vi "H3C psw cable 10G SFP+读写操作.vi"(6 "input_psw":u8[](array[numeric]) format="%.0x", 7 "input_psw 2":u8[](array[numeric]) format="%.0x", 8 "input_data":u8[](array[numeric]) format="%.0x", 9 "input_mode":string(combo), 10 "Channel":u8 max=5 step=1, 11 "VISA":refnum<visa-resource-name>="COM6") -> (0 "A2Hequal00?":bool, 1 "result":bool, 2 "message":string, 3 "data read":u8[](array[numeric]) format="%.0x")   [LabVIEW 2011]
panel:
  out "A2h后128个字节":u8[](array[numeric]) format="%.0x"
  out "A2h前128个字节":u8[](array[numeric]) format="%.0x"
  in  "address":u8
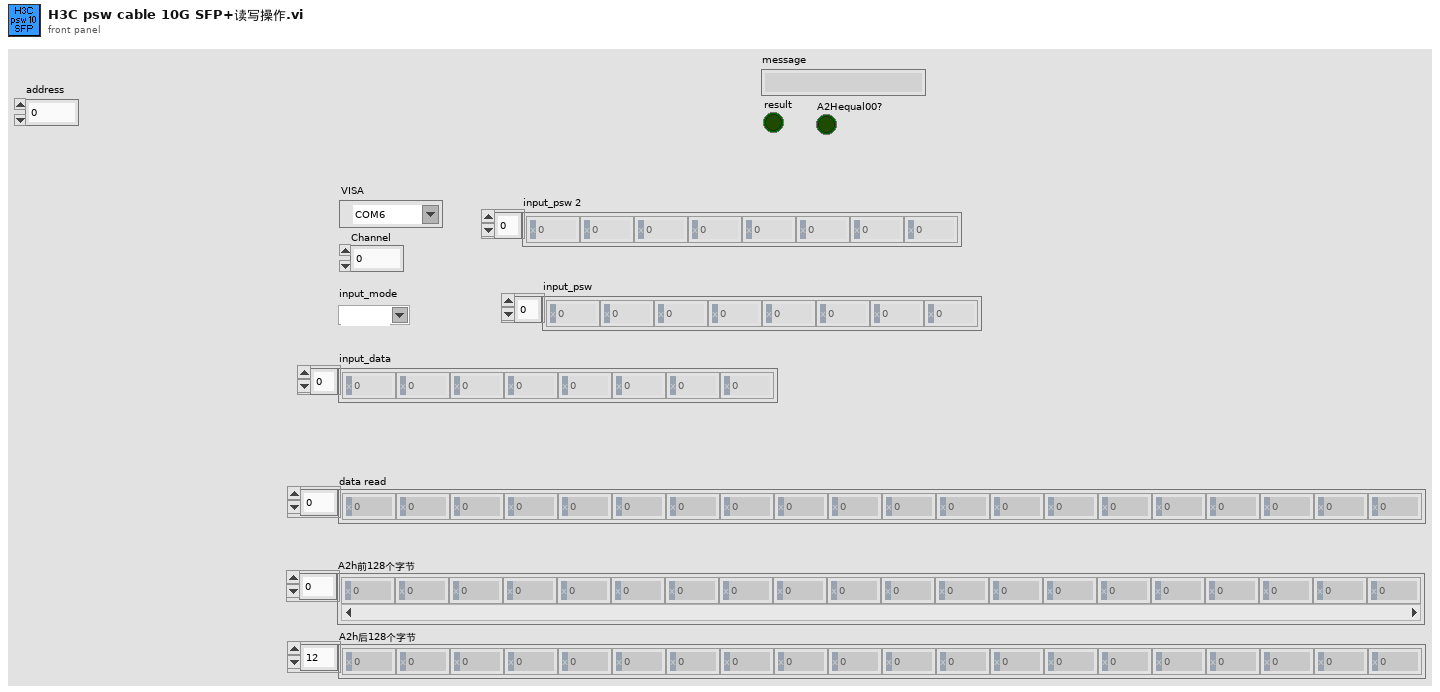
[diagram p1: front panel]
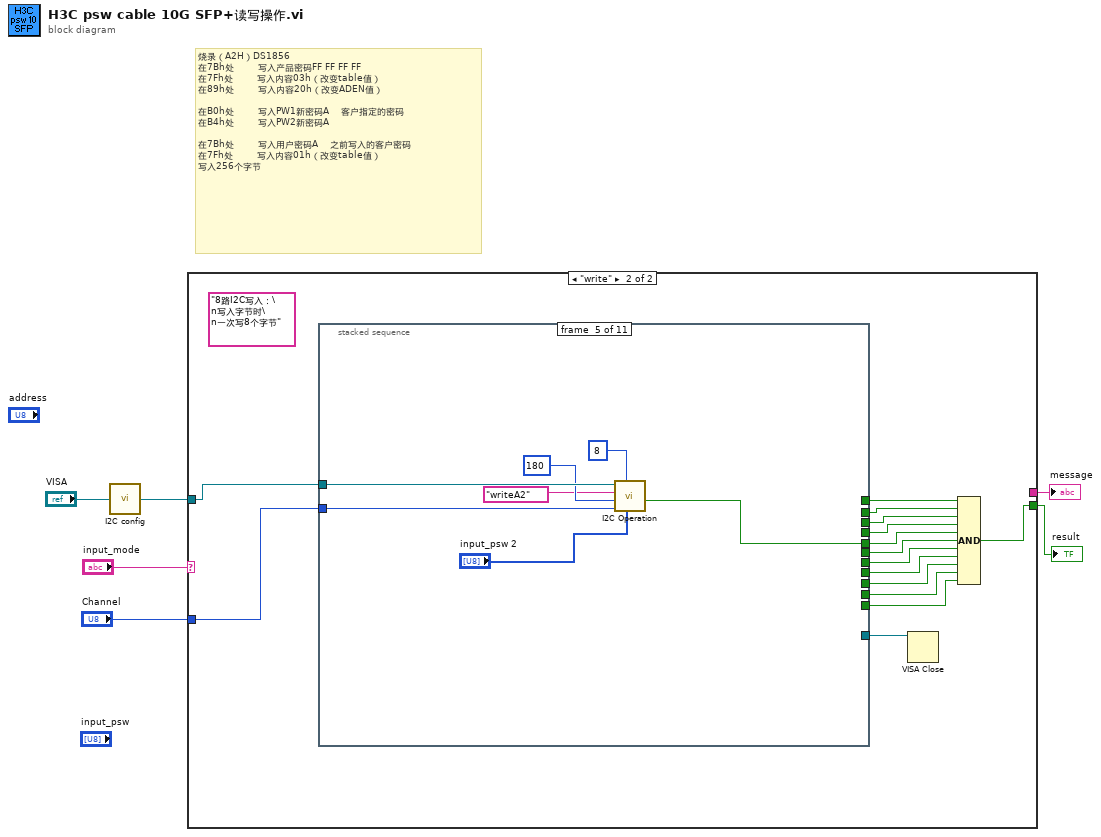
[diagram p0: block diagram]
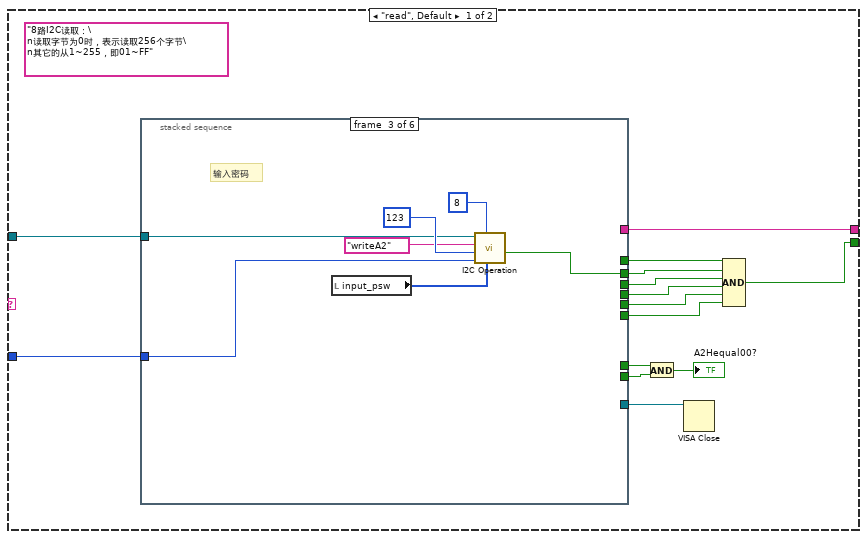
[diagram p2: hidden frame]
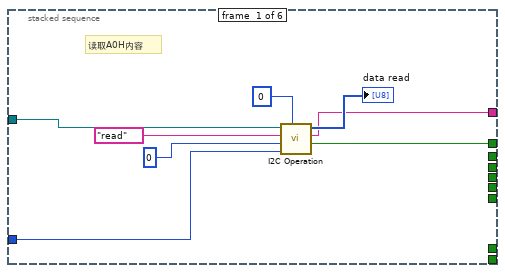
[diagram p3: hidden frame]
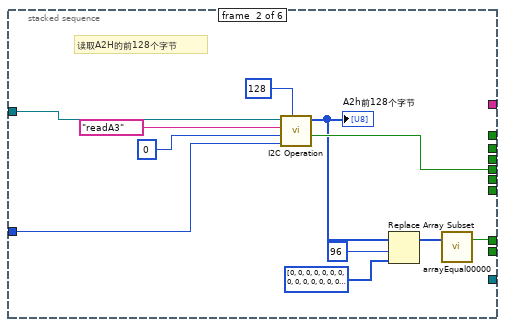
[diagram p4: hidden frame]
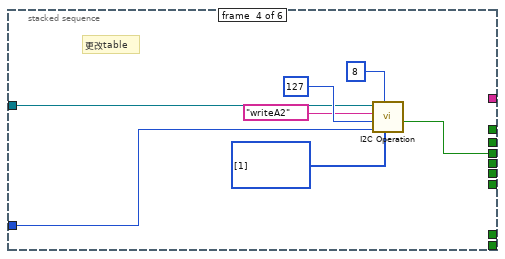
[diagram p5: hidden frame]
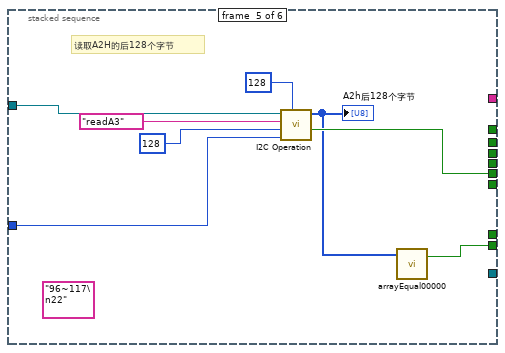
[diagram p6: hidden frame]
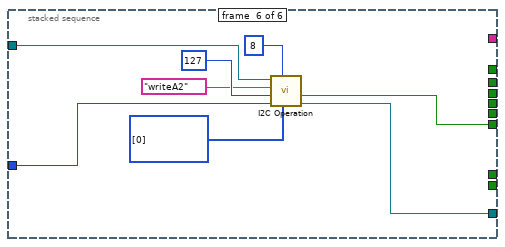
[diagram p7: hidden frame]
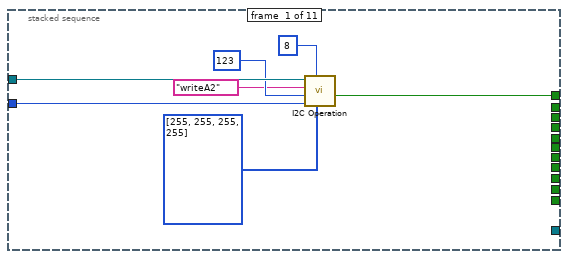
[diagram p8: hidden frame]
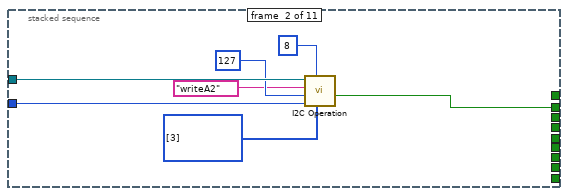
[diagram p9: hidden frame]
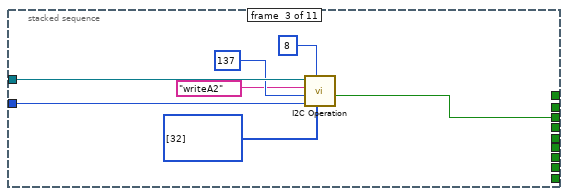
[diagram p10: hidden frame]
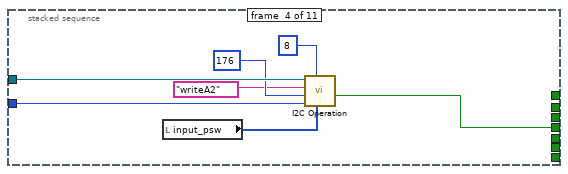
[diagram p11: hidden frame]
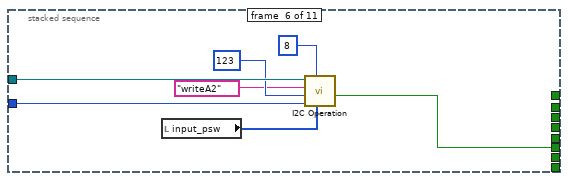
[diagram p12: hidden frame]
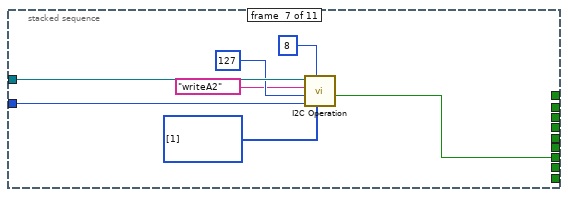
[diagram p13: hidden frame]
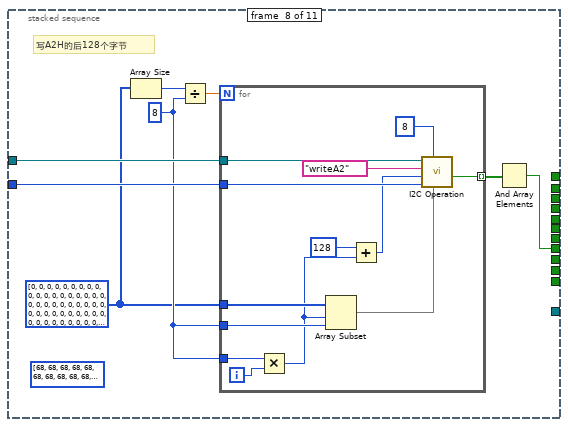
[diagram p14: hidden frame]
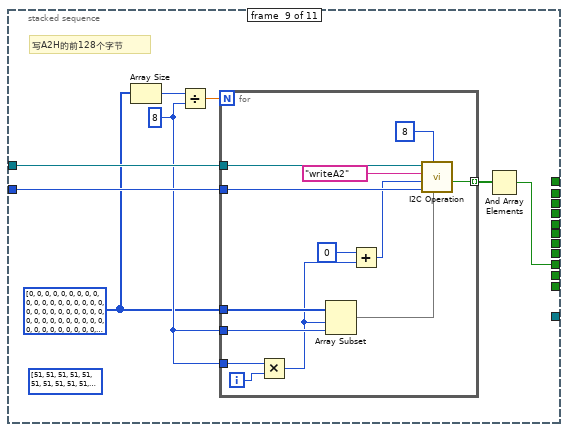
[diagram p15: hidden frame]
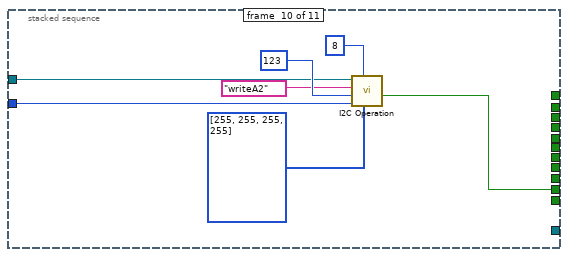
[diagram p16: hidden frame]
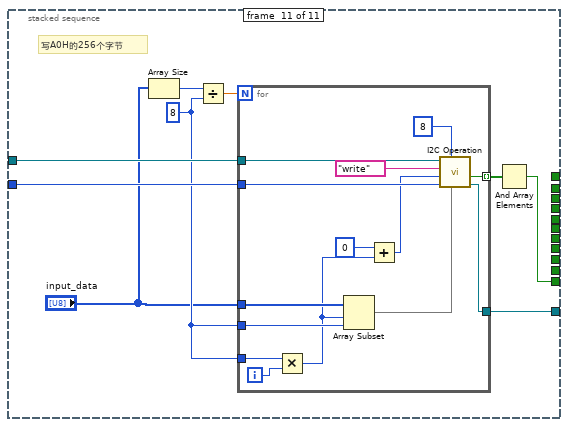
[diagram p17: hidden frame]
diagram:
  # "烧录（A2H）DS1856\n在7Bh处        写入产品密码FF FF FF FF\n在7Fh处        写入内容03h（改变table值）\n在89h处        写入内容20h（改变ADEN值）\n\n在B0h处        写入PW1新密码A    客户指定的密码\n在B4h处        写入PW2新密码A\n\n在7Bh处        写入用户密码A    之前写入的客户密码\n在7Fh处        写入内容01h（改变table值）\n写入256个字节"
  n1 = call "I2C config.vi"("VISA"="VISA") -> ("VISA资源名称输出"=w1:refnum<visa-resource-name>)
  n2 = case shown="\"write\"" "input_mode" {
    tunnel: w1 -> [w20 w84]
    tunnel: "Channel" -> [w19 w83]
    tunnel: [w18 _] -> w4
    tunnel: [w12 w71] -> w3
    frame "read", Default {
      (unwired) "8路I2C读取：\n读取字节为0时，表示读取256个字节\n其它的从1~255，即01~FF"
      n3 = stacked-sequence {
        tunnel: w20 -> [w28 w39 w42 w49 w61 w65]
        tunnel: w19 -> [w25 w36 w41 w48 w58 w64]
        tunnel: [w23 _ _ _ _ _] -> w18
        tunnel: [w22 _ _ _ _ _] -> w17
        tunnel: [_ _ w40 _ _ _] -> w16
        tunnel: [_ _ _ w47 _ _] -> w15
        tunnel: [_ w34 _ _ _ _] -> w14
        tunnel: [_ w33 _ _ _ _] -> w11
        tunnel: [_ _ _ _ w56 _] -> w13
        tunnel: [_ _ _ _ w55 _] -> w10
        tunnel: [_ _ _ _ _ w63] -> w8
        tunnel: [_ _ _ _ _ w62] -> w7
        frame #0 {
          # "读取A0H内容"
          n4 = call "I2C Operation.vi"("size"=0, "Channel"=w25, "address"=u8 0, "mode"="read", "VISA"=w28) -> ("result"=w22:bool, "message"=w23:string, "Data Out"=→"data read":u8[])  [unwired: 3 in, 1 out]
        }
        frame #1 {
          # "读取A2H的前128个字节"
          n5 = call "I2C Operation.vi"("size"=128, "Channel"=w36, "address"=u8 0, "mode"="readA3", "VISA"=w39) -> ("result"=w34:bool, "Data Out"=w29:u8[])  [unwired: 3 in, 2 out]
          "A2h前128个字节" <- w29
          n6 = Replace Array Subset(array=w29, new element=u8[] [0, 0, 0, 0, 0, 0, 0, 0, 0, 0, 0, 0, 0, 0, 0, 0, 0, 0, 0, 0, 0, 0], index=96 ("索引")) -> (w30:u8[])
          n7 = call "arrayEqual00000.vi"("input_array"=w30) -> ("show_bool_result"=w33:bool)  [unwired: 2 in]
        }
        frame #2 {
          # "输入密码"
          n8 = local read "input_psw"() -> (w44:u8[])
          n9 = call "I2C Operation.vi"("input_data"=w44, "size"=8, "Channel"=w41, "address"=u8 123, "mode"="writeA2", "VISA"=w42) -> ("result"=w40:bool)  [unwired: 2 in, 3 out]
        }
        frame #3 {
          # "更改table"
          n10 = call "I2C Operation.vi"("input_data"=u8[] [1], "size"=8, "Channel"=w48, "address"=u8 127, "mode"="writeA2", "VISA"=w49) -> ("result"=w47:bool)  [unwired: 2 in, 3 out]
        }
        frame #4 {
          (unwired) "96~117\n22"
          # "读取A2H的后128个字节"
          n11 = call "I2C Operation.vi"("size"=128, "Channel"=w58, "address"=u8 128, "mode"="readA3", "VISA"=w61) -> ("result"=w56:bool, "Data Out"=w54:u8[])  [unwired: 3 in, 2 out]
          "A2h后128个字节" <- w54
          n12 = call "arrayEqual00000.vi"("input_array"=w54) -> ("show_bool_result"=w55:bool)  [unwired: 2 in]
        }
        frame #5 {
          n13 = call "I2C Operation.vi"("input_data"=u8[] [0], "size"=8, "Channel"=w64, "address"=u8 127, "mode"="writeA2", "VISA"=w65) -> ("VISA  2"=w62:refnum<visa-resource-name>, "result"=w63:bool)  [unwired: 2 in, 2 out]
        }
      }
      n14 = And(x=w11, y=w10) -> (x .and. y?=→"A2Hequal00?":bool)
      n15 = VISA Close(VISA resource name=w7) -> ()  [unwired: 1 in, 1 out]
      n16 = Compound Arithmetic op=AND(w17, w16, w15, w14, w13, w8) -> (w12:bool)
    }
    frame "write" {
      (unwired) "8路I2C写入：\n写入字节时\n一次写8个字节"
      n17 = stacked-sequence {
        tunnel: w84 -> [w91 w98 w105 w112 w119 w126 w133 w141 w162 w179 w191]
        tunnel: w83 -> [w89 w96 w103 w110 w117 w124 w131 w140 w161 w178 w190]
        tunnel: [w85 _ _ _ _ _ _ _ _ _ _] -> w82
        tunnel: [_ w92 _ _ _ _ _ _ _ _ _] -> w81
        tunnel: [_ _ w99 _ _ _ _ _ _ _ _] -> w80
        tunnel: [_ _ _ w106 _ _ _ _ _ _ _] -> w79
        tunnel: [_ _ _ _ w114 _ _ _ _ _ _] -> w78
        tunnel: [_ _ _ _ _ w120 _ _ _ _ _] -> w77
        tunnel: [_ _ _ _ _ _ w127 _ _ _ _] -> w76
        tunnel: [_ _ _ _ _ _ _ w135 _ _ _] -> w75
        tunnel: [_ _ _ _ _ _ _ _ w156 _ _] -> w74
        tunnel: [_ _ _ _ _ _ _ _ _ w176 _] -> w73
        tunnel: [_ _ _ _ _ _ _ _ _ _ w185] -> w72
        tunnel: [_ _ _ _ _ _ _ _ _ _ w183] -> w70
        frame #0 {
          n18 = call "I2C Operation.vi"("input_data"=u8[] [255, 255, 255, 255], "size"=8, "Channel"=w89, "address"=u8 123, "mode"="writeA2", "VISA"=w91) -> ("result"=w85:bool)  [unwired: 2 in, 3 out]
        }
        frame #1 {
          n19 = call "I2C Operation.vi"("input_data"=u8[] [3], "size"=8, "Channel"=w96, "address"=u8 127, "mode"="writeA2", "VISA"=w98) -> ("result"=w92:bool)  [unwired: 2 in, 3 out]
        }
        frame #2 {
          n20 = call "I2C Operation.vi"("input_data"=u8[] [32], "size"=8, "Channel"=w103, "address"=u8 137, "mode"="writeA2", "VISA"=w105) -> ("result"=w99:bool)  [unwired: 2 in, 3 out]
        }
        frame #3 {
          n21 = local read "input_psw"() -> (w108:u8[])
          n22 = call "I2C Operation.vi"("input_data"=w108, "size"=8, "Channel"=w110, "address"=u8 176, "mode"="writeA2", "VISA"=w112) -> ("result"=w106:bool)  [unwired: 2 in, 3 out]
        }
        frame #4 {
          n23 = call "I2C Operation.vi"("input_data"="input_psw 2", "size"=8, "Channel"=w117, "address"=u8 180, "mode"="writeA2", "VISA"=w119) -> ("result"=w114:bool)  [unwired: 2 in, 3 out]
        }
        frame #5 {
          n24 = local read "input_psw"() -> (w122:u8[])
          n25 = call "I2C Operation.vi"("input_data"=w122, "size"=8, "Channel"=w124, "address"=u8 123, "mode"="writeA2", "VISA"=w126) -> ("result"=w120:bool)  [unwired: 2 in, 3 out]
        }
        frame #6 {
          n26 = call "I2C Operation.vi"("input_data"=u8[] [1], "size"=8, "Channel"=w131, "address"=u8 127, "mode"="writeA2", "VISA"=w133) -> ("result"=w127:bool)  [unwired: 2 in, 3 out]
        }
        frame #7 {
          (unwired) i32[] [68, 68, 68, 68, 68, 68, 68, 68, 68, 68, 68, 68, 68, 68, 68, 68, 68, 68, 68, 68, 68, 68, 68, 68, 68, 68, 68, 68, 68, 68, 68, 68, 68, 68, 68, 68, 68, 68, 68, 68, 68, 68, 68, 68, 68, 68, 68, 68, 68, 68, 68, 68, 68, 68, 68, 68, 68, 68, 68, 68, 68, 68, 68, 68, 68, 68, 68, 68, 68, 68, 68, 68, 68, 68, 68, 68, 68, 68, 68, 68, 68, 68, 68, 68, 68, 68, 68, 68, 68, 68, 68, 68, 68, 68, 68, 68, 68, 68, 68, 68, 68, 68, 68, 68, 68, 68, 68, 68, 68, 68, 68, 68, 68, 68, 68, 68, 68, 68, 68, 68, 68, 68, 68, 68, 68, 68, 68, 68]
          w137 = 8 ("y")
          w134 = u8[] [0, 0, 0, 0, 0, 0, 0, 0, 0, 0, 0, 0, 0, 0, 0, 0, 0, 0, 0, 0, 0, 0, 0, 0, 0, 0, 0, 0, 0, 0, 0, 0, 0, 0, 0, 0, 0, 0, 0, 0, 0, 0, 0, 0, 0, 0, 0, 0, 0, 0, 0, 0, 0, 0, 0, 0, 0, 0, 0, 0, 0, 0, 0, 0, 0, 0, 0, 0, 0, 0, 0, 0, 0, 0, 0, 0, 0, 0, 0, 0, 0, 0, 0, 0, 0, 0, 0, 0, 0, 0, 0, 0, 0, 0, 0, 0, 0, 0, 0, 0, 0, 0, 0, 0, 0, 0, 0, 0, 0, 0, 0, 0, 0, 0, 0, 0, 0, 0, 0, 0, 0, 0, 0, 0, 0, 0, 0, 0]
          # "写A2H的后128个字节"
          n27 = Array Size(array=w134) -> (size(s)=w139:i32)
          n28 = Divide(x=w139, y=w137) -> (x/y=w138:dbl)
          n29 = for {
            N: w138 -> [_]
            tunnel: w141 -> [w154]
            tunnel: w140 -> [w152]
            tunnel: w134 -> [w150]
            tunnel: w137 -> [w148]
            tunnel: w137 -> [w147]
            tunnel: [w142] -> w136 mode=indexing
            i -> [w149]
            n30 = Multiply(x=w148, y=w149) -> (x*y=w145:i32)
            n31 = Array Subset(array=w150, index=w145, length=w147) -> (w143:u8[])
            n32 = Add(x=u8 128 ("address"), y=w145) -> (x+y=w144:i32)
            n33 = call "I2C Operation.vi"("input_data"=w143, "size"=8, "Channel"=w152, "address"=w144, "mode"="writeA2", "VISA"=w154) -> ("result"=w142:bool)  [unwired: 2 in, 3 out]
          }
          n34 = And Array Elements(Boolean array=w136) -> (logical AND=w135:bool)
        }
        frame #8 {
          (unwired) i32[] [51, 51, 51, 51, 51, 51, 51, 51, 51, 51, 51, 51, 51, 51, 51, 51, 51, 51, 51, 51, 51, 51, 51, 51, 51, 51, 51, 51, 51, 51, 51, 51, 51, 51, 51, 51, 51, 51, 51, 51, 51, 51, 51, 51, 51, 51, 51, 51, 51, 51, 51, 51, 51, 51, 51, 51, 51, 51, 51, 51, 51, 51, 51, 51, 51, 51, 51, 51, 51, 51, 51, 51, 51, 51, 51, 51, 51, 51, 51, 51, 51, 51, 51, 51, 51, 51, 51, 51, 51, 51, 51, 51, 51, 51, 51, 51, 51, 51, 51, 51, 51, 51, 51, 51, 51, 51, 51, 51, 51, 51, 51, 51, 51, 51, 51, 51, 51, 51, 51, 51, 51, 51, 51, 51, 51, 51, 51, 51]
          w158 = 8 ("y")
          w155 = u8[] [0, 0, 0, 0, 0, 0, 0, 0, 0, 0, 0, 0, 0, 0, 0, 0, 0, 0, 0, 0, 0, 0, 0, 0, 0, 0, 0, 0, 0, 0, 0, 0, 0, 0, 0, 0, 0, 0, 0, 0, 0, 0, 0, 0, 0, 0, 0, 0, 0, 0, 0, 0, 0, 0, 0, 0, 0, 0, 0, 0, 0, 0, 0, 0, 0, 0, 0, 0, 0, 0, 0, 0, 0, 0, 0, 0, 0, 0, 0, 0, 0, 0, 0, 0, 0, 0, 0, 0, 0, 0, 0, 0, 0, 0, 0, 0, 0, 0, 0, 0, 0, 0, 0, 0, 0, 0, 0, 0, 0, 0, 0, 0, 0, 0, 0, 0, 0, 0, 0, 0, 0, 0, 0, 0, 0, 0, 0, 0]
          # "写A2H的前128个字节"
          n35 = Array Size(array=w155) -> (size(s)=w160:i32)
          n36 = Divide(x=w160, y=w158) -> (x/y=w159:dbl)
          n37 = for {
            N: w159 -> [_]
            tunnel: w162 -> [w175]
            tunnel: w161 -> [w173]
            tunnel: w155 -> [w171]
            tunnel: w158 -> [w169]
            tunnel: w158 -> [w168]
            tunnel: [w163] -> w157 mode=indexing
            i -> [w170]
            n38 = Multiply(x=w169, y=w170) -> (x*y=w166:i32)
            n39 = Array Subset(array=w171, index=w166, length=w168) -> (w164:u8[])
            n40 = Add(x=u8 0 ("address"), y=w166) -> (x+y=w165:i32)
            n41 = call "I2C Operation.vi"("input_data"=w164, "size"=8, "Channel"=w173, "address"=w165, "mode"="writeA2", "VISA"=w175) -> ("result"=w163:bool)  [unwired: 2 in, 3 out]
          }
          n42 = And Array Elements(Boolean array=w157) -> (logical AND=w156:bool)
        }
        frame #9 {
          n43 = call "I2C Operation.vi"("input_data"=u8[] [255, 255, 255, 255], "size"=8, "Channel"=w178, "address"=u8 123, "mode"="writeA2", "VISA"=w179) -> ("result"=w176:bool)  [unwired: 2 in, 3 out]
        }
        frame #10 {
          w187 = 8 ("y")
          # "写A0H的256个字节"
          n44 = Array Size(array="input_data") -> (size(s)=w189:i32)
          n45 = Divide(x=w189, y=w187) -> (x/y=w188:dbl)
          n46 = for {
            N: w188 -> [_]
            tunnel: w191 -> [w205]
            tunnel: w190 -> [w203]
            tunnel: "input_data" -> [w201]
            tunnel: w187 -> [w199]
            tunnel: w187 -> [w198]
            tunnel: [w193] -> w186 mode=indexing
            tunnel: [w192] -> w183
            i -> [w200]
            n47 = Multiply(x=w199, y=w200) -> (x*y=w196:i32)
            n48 = Array Subset(array=w201, index=w196, length=w198) -> (w194:u8[])
            n49 = Add(x=u8 0 ("address"), y=w196) -> (x+y=w195:i32)
            n50 = call "I2C Operation.vi"("input_data"=w194, "size"=8, "Channel"=w203, "address"=w195, "mode"="write", "VISA"=w205) -> ("VISA  2"=w192:refnum<visa-resource-name>, "result"=w193:bool)  [unwired: 2 in, 2 out]
          }
          n51 = And Array Elements(Boolean array=w186) -> (logical AND=w185:bool)
        }
      }
      n52 = VISA Close(VISA resource name=w70) -> ()  [unwired: 1 in, 1 out]
      n53 = Compound Arithmetic op=AND(w82, w81, w80, w79, w78, w77, w76, w75, w74, w73, w72) -> (w71:bool)
    }
  }
  "message" <- w4
  "result" <- w3
